vi "SMO.UI.GetPrivateEvents.vi"(8 "error in (no error)":errorcluster, 11 "SMO.UI":refnum<class "SMO.UI.lvclass">) -> (0 "error out":errorcluster, 2 "SMO.UI Private Events":T1, 3 "SMO.UI out":refnum<class "SMO.UI.lvclass">)   [LabVIEW 2021, in "smo.lvlib" / "SMO.UI.lvclass"]
uses:
  SMO.UI.lvclass
  Typedefs/PrivateEvents--Cluster.ctl
  SMO.UI.lvclass/SMO.UI.ctl
panel:
  # "For instructions on how to use the JKI State Machine Objects, examples and video tutorials, visit:\nhttp://jki.net/state-machine-objects/\n\nJKI State Machine Objects™\nhttp://jki.net/state-machine-objects/\nCopyright (C) 2005-2015, JKI <info@jki.net>\nALL RIGHTS RESERVED"
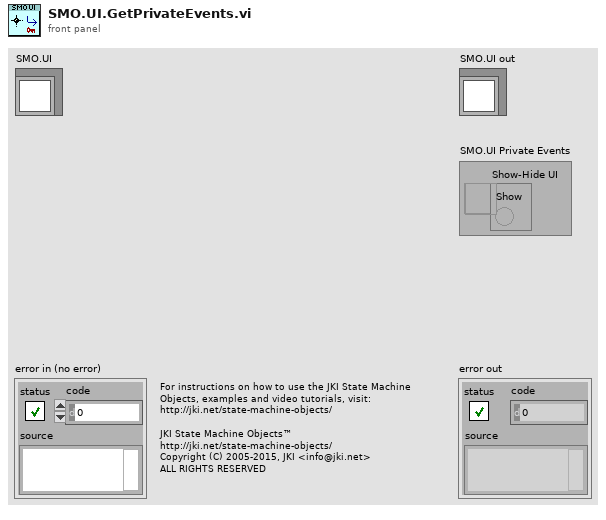
[diagram p1: front panel]
types:
  T1 = typedef "smo.lvlib/SMO.UI.lvclass/PrivateEvents--Cluster.ctl" = cluster{"Show-Hide UI":refnum<user-event>}
  T2 = typedef "smo.lvlib/SMO.UI.lvclass/PrivateData--Ref.ctl" = refnum<data-value>
  T3 = typedef "smo.lvlib/SMO.UI.lvclass/PrivateData--Cluster.ctl" = cluster{"Public Events":T4, "Private Events":T1}
  T4 = typedef "smo.lvlib/SMO.UI.lvclass/PublicEvents--Cluster.ctl" = cluster{"UI Hidden":refnum<user-event>, "UI State":refnum<user-event>}
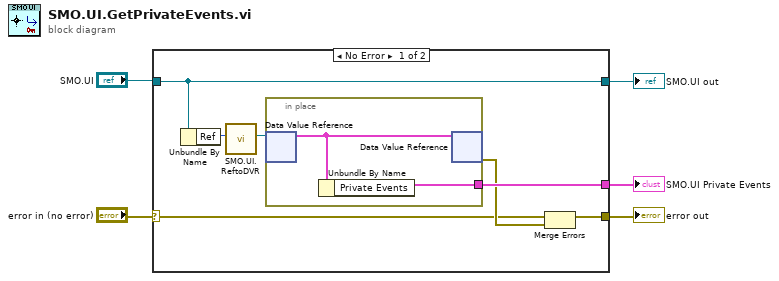
[diagram p0: block diagram]
diagram:
  n1 = case shown="No Error" "error in (no error)" {
    selector: "error in (no error)" -> [w6 w16]
    tunnel: [w12 w16] -> w2
    tunnel: [w7 w15] -> w4
    tunnel: "SMO.UI" -> [w7 w15]
    tunnel: [w11 _] -> w1
    frame No Error {
      n2 = Unbundle By Name(w7) -> ("Ref"=w9:u32)
      n3 = call "SMO.UI.ReftoDVR.vi"("Ref"=w9) -> ("Ref"=w8:T2)  [unwired: 10 in]
      n4 = in-place {
        in-place-border: [w14] -> w11
        n5 = in-place-dvr #1(w8) -> (w13:T3)  [unwired: 1 out]
        n6 = Unbundle By Name(w13) -> ("Private Events"=w14:T1)
        n7 = in-place-dvr #1(w13) -> (w10:errorcluster)  [unwired: 1 out]
      }
      n8 = Merge Errors(w6, w10) -> (w12:errorcluster)
    }
    frame Error {
    }
  }
  "error out" <- w2
  "SMO.UI out" <- w4
  "SMO.UI Private Events" <- w1
